vi "Digital_In.vi"(6 "Waveform_Template":waveform(dbl), 8 "error in":errorcluster, 11 "DAQ970 in":refnum<class "DAQ970.lvclass">) -> (0 "error out":errorcluster, 2 "DC_Voltage_Measurement":waveform(dbl)[](array[waveform]), 3 "DAQ970 out":refnum<class "DAQ970.lvclass">)   [LabVIEW 2019, in "DAQ970.lvlib" / "DAQ970.lvclass"]
uses:
  Library/DAQ970.lvclass
  Library/DAQ970.lvclass/DAQ970.ctl
  <instrlib>/Keysight DAQ970/Keysight DAQ970.lvlib
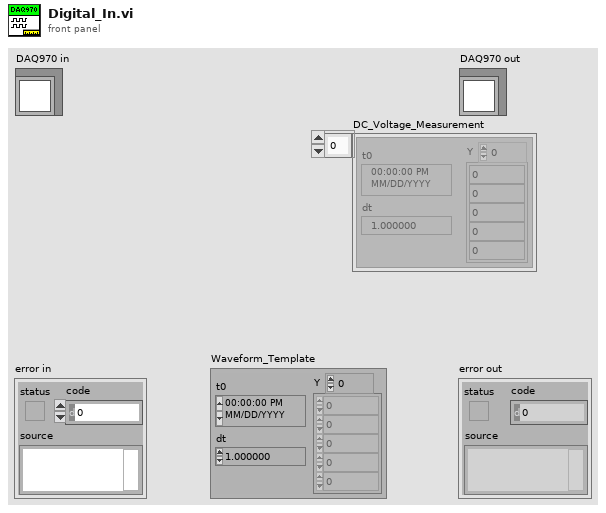
[diagram p1: front panel]
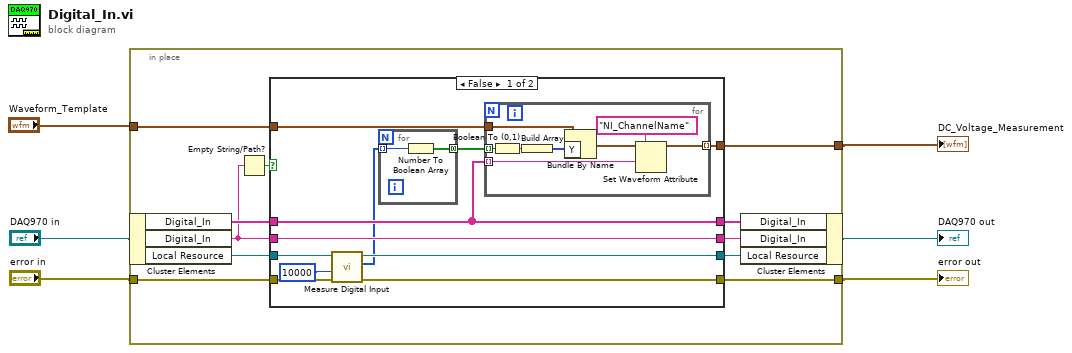
[diagram p0: block diagram]
diagram:
  n1 = in-place {
    in-place-border: "error in" -> [w11]
    in-place-border: [w12] -> w2
    in-place-border: "Waveform_Template" -> [w17]
    in-place-border: [w15] -> w6
    n2 = in-place-cluster #1("DAQ970 in") -> ("Digital_In"=w16:string[], "Digital_In"=w10:string, "Local Resource"=w14:refnum<k15>)
    n3 = Empty String/Path?(string/path=w10) -> (empty?=w9:bool)
    n4 = case shown="False" w9 {
      tunnel: w17 -> [w28 _]
      tunnel: w16 -> [w26 w42]
      tunnel: [w27 _] -> w15
      tunnel: w14 -> [w24 w40]
      tunnel: [w23 w40] -> w13
      tunnel: [w22 w39] -> w12
      tunnel: w11 -> [w21 w39]
      tunnel: w10 -> [w25 w41]
      tunnel: [w26 w42] -> w8
      tunnel: [w25 w41] -> w7
      frame False {
        n5 = call <instrlib>:"Measure Digital Input.vi"("error in (no error)"=w21, "MaxTimeMilliseconds"=10000, "instrument handle"=w24) -> ("error out"=w22:errorcluster, "Val"=w19:i32[], "instrument handle out"=w23:refnum<k15>)  [unwired: 5 in, 1 out]
        n6 = for {
          tunnel: w19 -> [w30] mode=indexing
          tunnel: [w29] -> w18 mode=concatenating
          n7 = Number To Boolean Array(number=w30) -> (Boolean array=w29:bool[])
        }
        n8 = for {
          tunnel: w18 -> [w37] mode=indexing
          tunnel: w28 -> [w38]
          tunnel: w26 -> [w34] mode=indexing
          tunnel: [w33] -> w27 mode=indexing
          n9 = Boolean To (0,1)(Boolean=w37) -> (0, 1=w31:i16)
          n10 = Build Array(w31) -> (w32:i16[])
          n11 = Bundle By Name(cluster=w38, "Y"=w32) -> (w36:waveform(dbl))
          n12 = Set Waveform Attribute(5:w34, 6:"NI_ChannelName" ("name"), 7:w36) -> (3:w33:waveform(dbl))  [unwired: 1 in, 2 out]
        }
      }
      frame True {
      }
    }
    n13 = in-place-cluster #1("Digital_In"=w8, "Digital_In"=w7, "Local Resource"=w13) -> (→"DAQ970 out":refnum<class "DAQ970.lvclass">)
  }
  "error out" <- w2
  "DC_Voltage_Measurement" <- w6
